vi "UI - Initialize IO Variables.vi"(8 "error in (no error)":errorcluster, 11 "Controller Address":string) -> (0 "error out":errorcluster, 3 "IO References":T1)   [LabVIEW 2017]
uses:
  controls/IO References.ctl
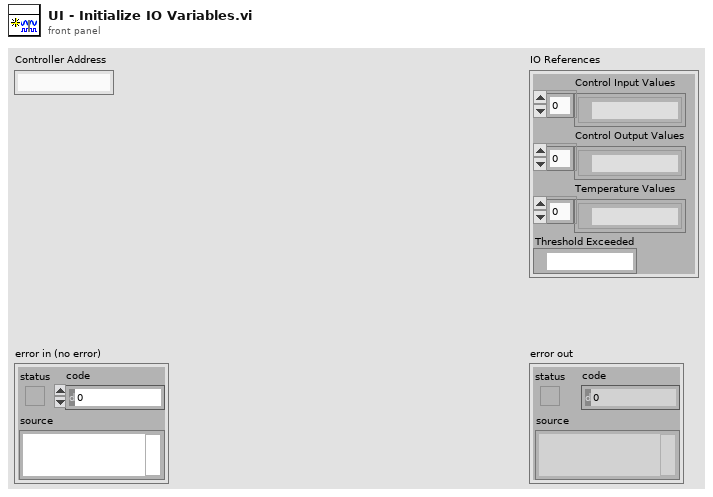
[diagram p1: front panel]
types:
  T1 = typedef "IO References.ctl" = cluster{"Control Input Values":refnum<k21>[], "Control Output Values":refnum<k21>[], "Temperature Values":refnum<k21>[], "Threshold Exceeded":refnum<k21>}
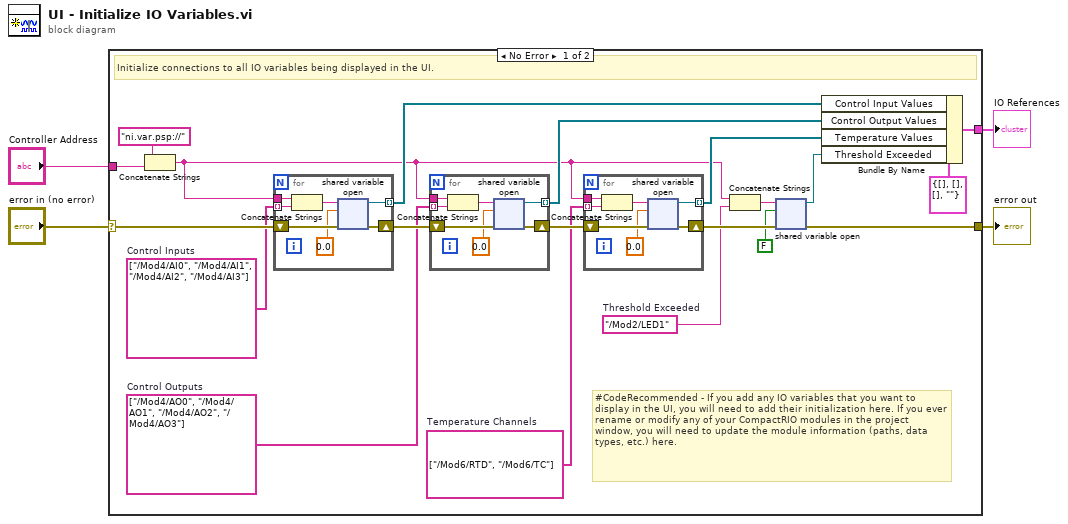
[diagram p0: block diagram]
diagram:
  n1 = case shown="No Error" "error in (no error)" {
    selector: "error in (no error)" -> [w21 w46]
    tunnel: "Controller Address" -> [w23 _]
    tunnel: [w6 w46] -> w2
    tunnel: [w18 _] -> w1
    frame No Error {
      w5 = string[] ["/Mod6/RTD", "/Mod6/TC"]  # Temperature Channels
      w10 = "/Mod2/LED1"  # Threshold Exceeded
      w16 = string[] ["/Mod4/AO0", "/Mod4/AO1", "/Mod4/AO2", "/Mod4/AO3"]  # Control Outputs
      w20 = string[] ["/Mod4/AI0", "/Mod4/AI1", "/Mod4/AI2", "/Mod4/AI3"]  # Control Inputs
      # "#CodeRecommended - If you add any IO variables that you want to display in the UI, you will need to add their initialization here. If you ever rename or modify any of your CompactRIO modules in the project window, you will need to update the module information (paths, data types, etc.) here."
      # "Initialize connections to all IO variables being displayed in the UI."
      n2 = Concatenate Strings("ni.var.psp://", w23) -> (w12:string)
      n3 = for {
        shift-right: [w44] -> w17
        shift-left: w21 -> [w45]
        tunnel: w12 -> [w41]
        tunnel: w20 -> [w40] mode=indexing
        tunnel: [w39] -> w19 mode=indexing
        n4 = Concatenate Strings(w41, w40) -> (w43:string)
        n5 = shared-variable-open(w43, w45, 0.0) -> (w39:refnum<k21>, w44:errorcluster)  [unwired: 1 in]
      }
      n6 = for {
        shift-right: [w37] -> w14
        shift-left: w17 -> [w38]
        tunnel: w12 -> [w34]
        tunnel: w16 -> [w33] mode=indexing
        tunnel: [w32] -> w15 mode=indexing
        n7 = Concatenate Strings(w34, w33) -> (w36:string)
        n8 = shared-variable-open(w36, w38, 0.0) -> (w32:refnum<k21>, w37:errorcluster)  [unwired: 1 in]
      }
      n9 = for {
        shift-right: [w30] -> w11
        shift-left: w14 -> [w31]
        tunnel: w12 -> [w27]
        tunnel: w5 -> [w26] mode=indexing
        tunnel: [w25] -> w13 mode=indexing
        n10 = Concatenate Strings(w27, w26) -> (w29:string)
        n11 = shared-variable-open(w29, w31, 0.0) -> (w25:refnum<k21>, w30:errorcluster)  [unwired: 1 in]
      }
      n12 = Concatenate Strings(w12, w10) -> (w9:string)
      n13 = shared-variable-open(w9, w11, FALSE) -> (w7:refnum<k21>, w6:errorcluster)  [unwired: 1 in]
      n14 = Bundle By Name(cluster=T1 {"Control Input Values"=[], "Control Output Values"=[], "Temperature Values"=[], "Threshold Exceeded"=""} ("IO References"), "Control Input Values"=w19, "Control Output Values"=w15, "Temperature Values"=w13, "Threshold Exceeded"=w7) -> (w18:T1)
    }
    frame Error {
      # "Error"
    }
  }
  "error out" <- w2
  "IO References" <- w1
